vi "SrvSetMask.vi"(0 "ref in":u64, 7 "Mask":u32, 11 "error in (no error)":errorcluster) -> (4 "ref out":u64, 8 "return type":i32, 15 "error out":errorcluster)   [LabVIEW 2019, in "Snap7.lvlib"]
uses:
  Snap7.lvlib
  windows/lv_snap7.dll
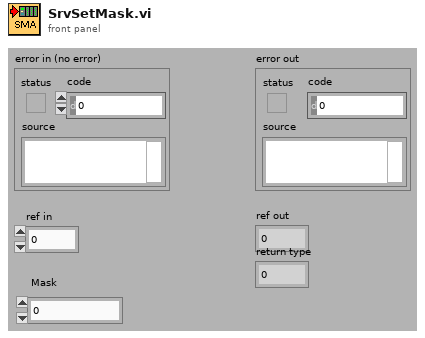
[diagram p1: front panel]
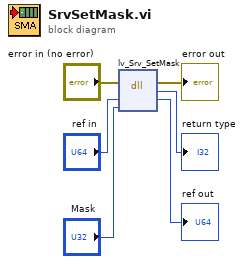
[diagram p0: block diagram]
diagram:
  n1 = dll-call lib="PTH2Xabs DSVNHLCEPStrunk性能试验台SourcesSnap7libwindowslv_snap7.dll" fn="lv_Srv_SetMask"(error in="error in (no error)", "Server"="ref in", "Mask"="Mask") -> (error out=→"error out":errorcluster, "return type"=→"return type":i32, "Server"=→"ref out":u64)  [unwired: 3 in, 1 out]
